vi "Host Event Log.vi"(6 "Operation":enum16{"Create", "Write", "Close", "Header"}(ring)=enum."Write", 7 "Event":string, 8 "error in":errorcluster, 10 "Enable":bool=TRUE) -> (0 "error out":errorcluster)   [LabVIEW 2021]
uses:
  <vilib>/Utility/sysdir.llb/System Directory Type.ctl
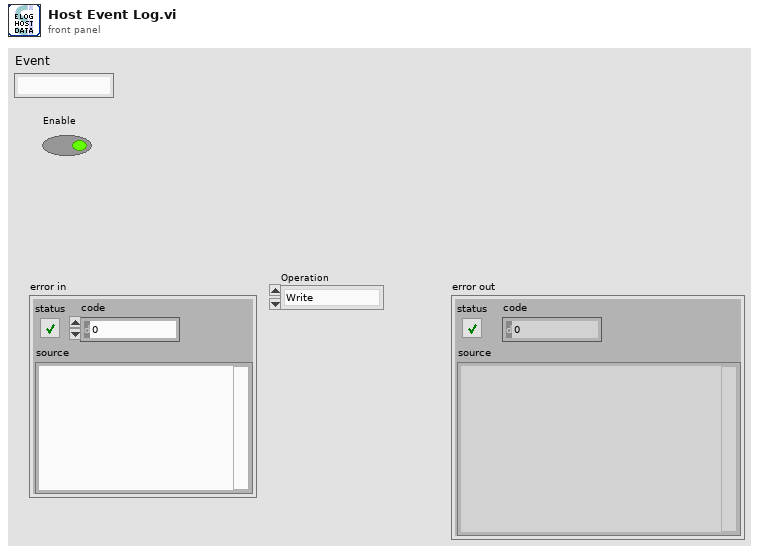
[diagram p1: front panel]
types:
  T1 = enum16{"open", "replace", "create", "open or create", "replace or create", "replace or create with confirmation"}
  T2 = typedef "System Directory Type.ctl" = i32
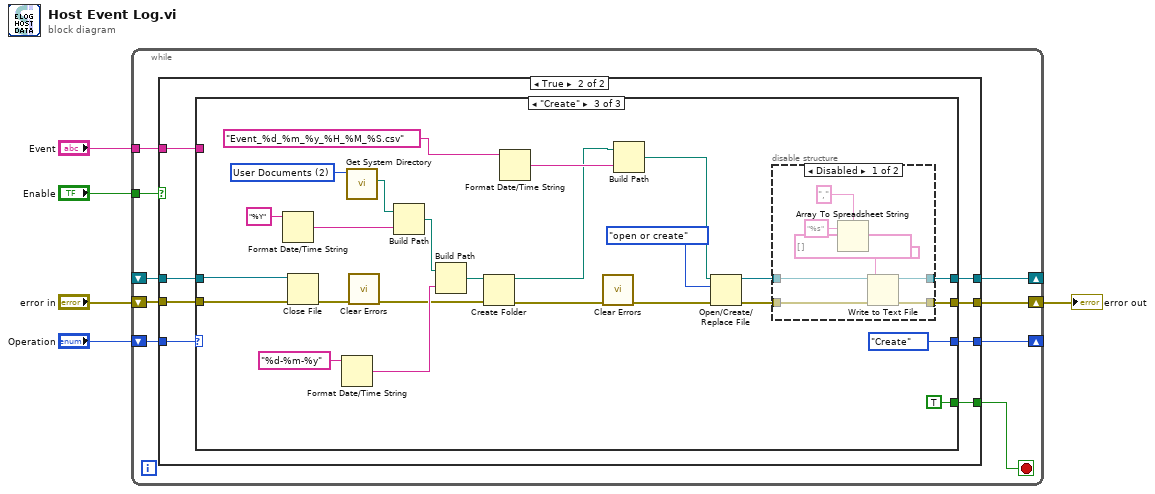
[diagram p0: block diagram]
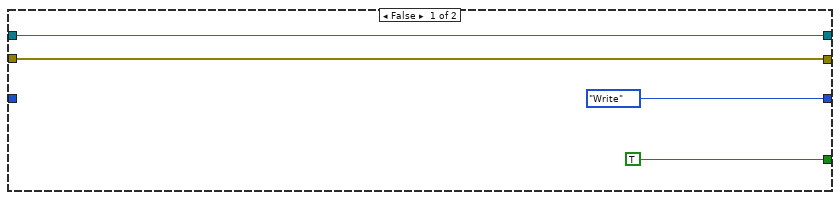
[diagram p2: hidden frame]
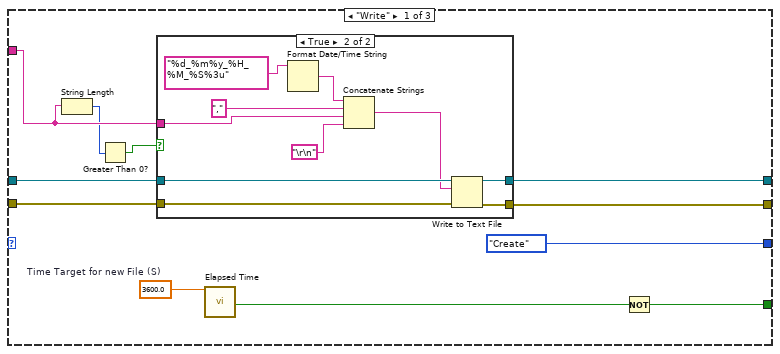
[diagram p3: hidden frame]
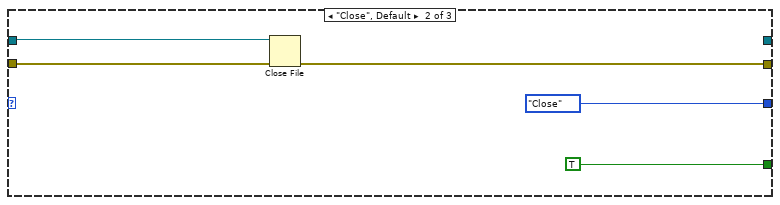
[diagram p5: hidden frame]
diagram:
  n1 = while {
    shift-right: [w13] -> _
    shift-left: _ -> [w12]
    shift-right: [w11] -> w3
    shift-left: "error in" -> [w10]
    tunnel: "Enable" -> [w9]
    shift-right: [w7] -> _
    shift-left: "Operation" -> [w14]
    tunnel: "Event" -> [w6]
    stop <- w8 stop-if-true
    n2 = case shown="True" w9 {
      tunnel: w14 -> [_ w26]
      tunnel: [w18 w25] -> w13
      tunnel: w12 -> [w18 w24]
      tunnel: [w17 w23] -> w11
      tunnel: w10 -> [w17 w22]
      tunnel: [TRUE w21] -> w8
      tunnel: [enum16{"Create", "Write", "Close"}."Write" ("Operation 2") w20] -> w7
      tunnel: w6 -> [_ w19]
      frame False {
      }
      frame True {
        n3 = case shown="\"Create\"" w26 {
          tunnel: [w36 _ w57] -> w25
          tunnel: w24 -> [w32 w52 w63]
          tunnel: [w37 w53 w59] -> w23
          tunnel: w22 -> [w33 w54 w65]
          tunnel: [w30 TRUE TRUE] -> w21
          tunnel: [enum16{"Create", "Write", "Close", "Header"}."Create" ("Operation") enum16{"Create", "Write", "Close"}."Close" ("Operation 2") enum16{"Create", "Write", "Close", "Header"}."Create" ("Operation")] -> w20
          tunnel: w19 -> [w29 _ _]
          frame "Write" {
            w34 = 3600.0  # Time Target for new File (S)
            n4 = String Length(string=w29) -> (length=w28:i32)
            n5 = Greater Than 0?(x=w28) -> (x > 0?=w27:bool)
            n6 = case shown="True" w27 {
              tunnel: [w38 w49] -> w37
              tunnel: [w39 w48] -> w36
              tunnel: w33 -> [w38 w47]
              tunnel: w32 -> [w39 w46]
              tunnel: w29 -> [_ w41]
              frame False {
              }
              frame True {
                n7 = Format Date/Time String(time format string (%c)="%d_%m%y_%H_%M_%S%3u") -> (date/time string=w45:string)  [unwired: 2 in]
                n8 = Concatenate Strings(w45, "," ("delimiter (Tab)"), w41, "\r\n") -> (w40:string)
                n9 = Write to Text File(file (use dialog)=w46, text=w40, error in=w47) -> (refnum out=w48:refnum<file>, error out=w49:errorcluster)  [unwired: 1 in, 1 out]
              }
            }
            n10 = call "Elapsed Time"("Time Target (s)"=w34) -> ("Time has Elapsed"=w35:bool)  [unwired: 11 in, 7 out]
            n11 = Not(x=w35) -> (.not. x?=w30:bool)
          }
          frame "Close", Default {
            n12 = Close File(refnum=w52, error in=w54) -> (error out=w53:errorcluster)  [unwired: 1 out]
          }
          frame "Create" {
            w79 = T2 2 items=["User Home"=0, "User Desktop"=1, "User Documents"=2, "User Application Data"=3, "User Preferences"=4, "User Temporary"=5, "Public Documents"=6, "Public Application Data"=7, "Public Preferences"=8, "Public Cache"=13, "System Core Libraries"=9, "System Installed Libraries"=10, "Application Files"=11, "Boot Volume Root"=12] ("system directory type")
            n13 = Format Date/Time String(time format string (%c)="%Y") -> (date/time string=w75:string)  [unwired: 2 in]
            n14 = Close File(refnum=w63, error in=w65) -> (error out=w64:errorcluster)  [unwired: 1 out]
            n15 = Format Date/Time String(time format string (%c)="%d-%m-%y") -> (date/time string=w73:string)  [unwired: 2 in]
            n16 = call <vilib>:"Get System Directory.vi"("system directory type"=w79) -> ("system directory"=w76:path)  [unwired: 10 in]
            n17 = call <vilib>:"Clear Errors.vi"("error in (no error)"=w64) -> ("error out"=w62:errorcluster)  [unwired: 5 in, 1 out]
            n18 = Build Path(base path=w76, name or relative path=w75) -> (appended path=w74:path)
            n19 = Build Path(base path=w74, name or relative path=w73) -> (appended path=w67:path)
            n20 = Create Folder(path (use dialog)=w67, error in=w62) -> (created path=w55:path, error out=w56:errorcluster)  [unwired: 1 in, 1 out]
            n21 = Format Date/Time String(time format string (%c)="Event_%d_%m_%y_%H_%M_%S.csv") -> (date/time string=w71:string)  [unwired: 2 in]
            n22 = call <vilib>:"Clear Errors.vi"("error in (no error)"=w56) -> ("error out"=w68:errorcluster)  [unwired: 5 in, 1 out]
            n23 = Build Path(base path=w55, name or relative path=w71) -> (appended path=w69:path)
            n24 = Open/Create/Replace File(file path (use dialog)=w69, error in=w68, operation (0:open)=T1."open or create") -> (refnum out=w58:refnum<file>, error out=w60:errorcluster)  [unwired: 3 in, 1 out]
            n25 = disable-structure shown="Disabled" {
              disable-tunnel: w60 -> [w84 w88]
              disable-tunnel: [w83 w88] -> w59
              disable-tunnel: w58 -> [w82 w89]
              disable-tunnel: [w81 w89] -> w57
              frame Disabled {
                n26 = Array To Spreadsheet String(delimiter (Tab)=",", array=string[] [], 3:"%s" ("format string")) -> (spreadsheet string=w87:string)
                n27 = Write to Text File(file (use dialog)=w82, text=w87, error in=w84) -> (refnum out=w81:refnum<file>, error out=w83:errorcluster)  [unwired: 1 in, 1 out]
              }
              frame Enabled {
              }
            }
          }
        }
      }
    }
  }
  "error out" <- w3
